vi "stage_get_status.vi"(8 "error in (no error)":errorcluster, 10 "Stage Name":string, 11 "Stage in":refnum<class "thorlabs_kinesis.lvclass">) -> (0 "error out":errorcluster, 2 "Status":string, 3 "Stage out":refnum<class "thorlabs_kinesis.lvclass">)   [LabVIEW 2015, in "thorlabs_kinesis.lvclass"]
uses:
  thorlabs_kinesis.lvclass
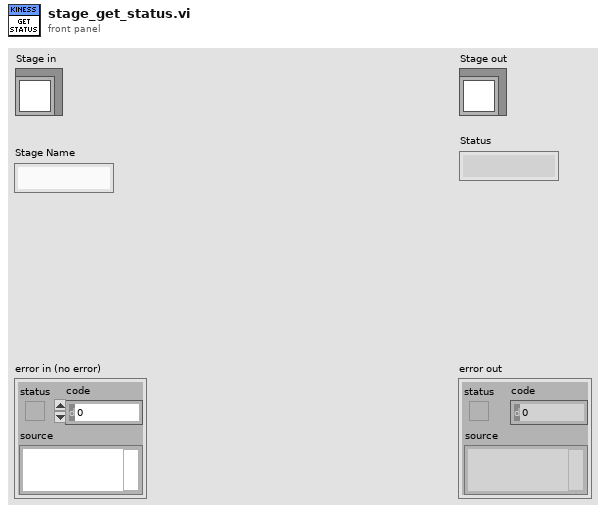
[diagram p1: front panel]
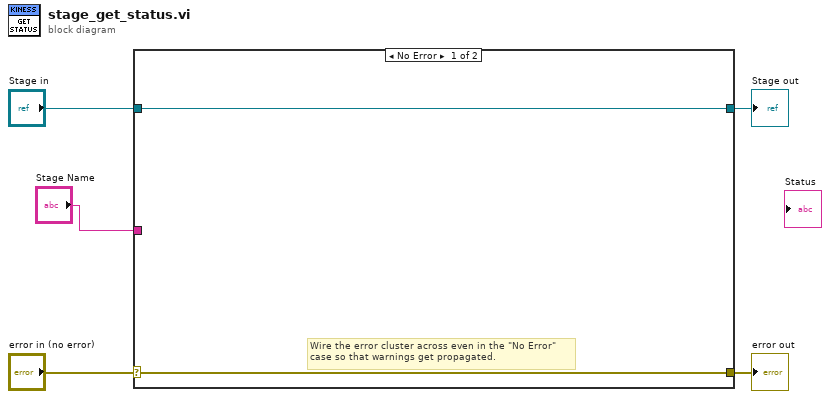
[diagram p0: block diagram]
diagram:
  n1 = case shown="No Error" "error in (no error)" {
    selector: "error in (no error)" -> [w6 w9]
    tunnel: [w6 w9] -> w4
    tunnel: [w7 w8] -> w2
    tunnel: "Stage in" -> [w7 w8]
    tunnel: "Stage Name" -> [_ _]
    frame No Error {
      # "Wire the error cluster across even in the \"No Error\"\ncase so that warnings get propagated."
    }
    frame Error {
    }
  }
  "error out" <- w4
  "Stage out" <- w2
